vi "DC Motor Control V1.vi"() -> ()   [LabVIEW 2013, in "LabVIEW Interface for Arduino.lvlib"]
doc: "An example that reads a user selectable analog input pin on the Arduino."
uses:
  <vilib>/LabVIEW Interface for Arduino/LabVIEW Interface for Arduino.lvlib
  <vilib>/LabVIEW Interface for Arduino/Type Defs/Pin Mode.ctl
panel:
  in  "PWM1 Pin":u8
  in  "Stop":bool
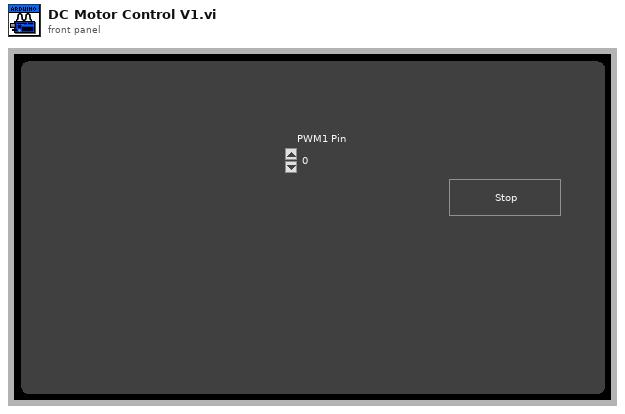
[diagram p1: front panel]
types:
  T1 = typedef "LabVIEW Interface for Arduino.lvlib/Pin Mode.ctl" = enum8{"Input", "Output"}
  T2 = typedef "LabVIEW Interface for Arduino.lvlib/Arduino Resource.ctl" = cluster{"VISA resource":refnum<visa-resource-name>, "Board Type":T3, "Connection Type":enum8{"USB / Serial"}, "Bytes Per Packet (15)":u8}
  T3 = typedef "LabVIEW Interface for Arduino.lvlib/Board Type.ctl" = enum16{"Uno", "Dimuelanove w/Atmega 328", "Mega 2560"}
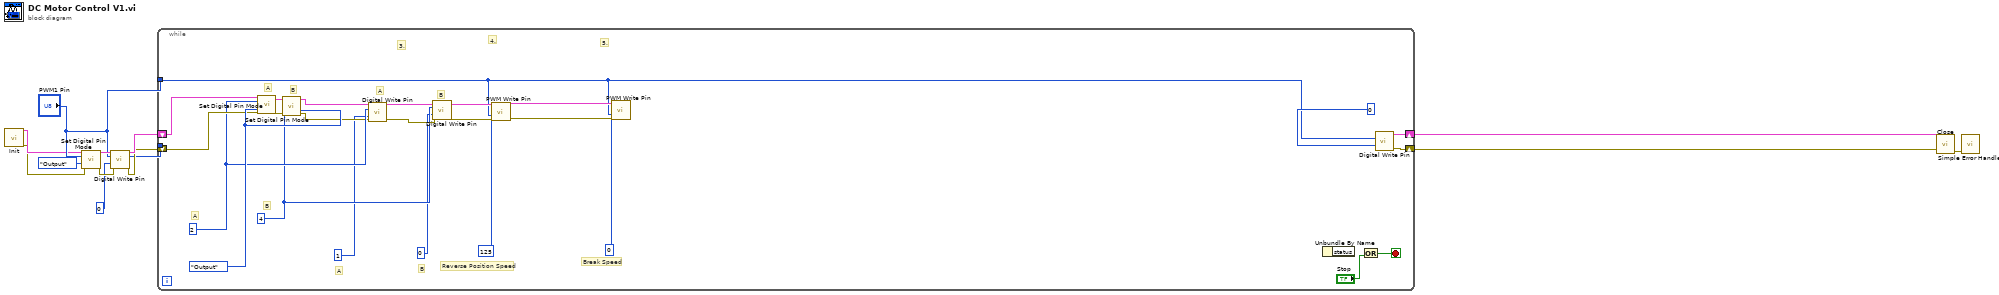
[diagram p0: block diagram]
diagram:
  n1 = call <vilib>:"Init.vi"() -> ("Arduino Resource"=w3:T2, "error out"=w2:errorcluster)  [unwired: 18 in]
  n2 = call <vilib>:"Set Digital Pin Mode.vi"("Arduino Resource"=w3, "Digital I/O Pin"="PWM1 Pin", "Pin Mode (Input)"=Pin_Mode."Output", "error in"=w2) -> ("Arduino Resource"=w9:T2, "error out"=w8:errorcluster)  [unwired: 10 in]
  n3 = call <vilib>:"Digital Write Pin.vi"("Arduino Resource"=w9, "Digital I/O Pin (0)"="PWM1 Pin", "Value (0)"=u8 0, "error in"=w8) -> ("Arduino Resource"=w6:T2, "error out"=w5:errorcluster)  [unwired: 10 in]
  n4 = while {
    shift-right: [w34] -> w11
    shift-left: w6 -> [w27]
    shift-right: [w33] -> w10
    shift-left: w5 -> [w26]
    tunnel: "PWM1 Pin" -> [_]
    tunnel: "PWM1 Pin" -> [w13]
    stop <- w37 stop-if-true
    w24 = u8 4 ("Digital I/O Pin")
    w25 = u8 2 ("Digital I/O Pin")
    w32 = Pin_Mode."Output" ("Pin Mode (Input)")
    # "Break Speed"
    # "5."
    # "4."
    # "Reverse Position Speed"
    # "3."
    # "B"
    # "A"
    # "B"
    # "A"
    # "B"
    # "A"
    # "B"
    # "A"
    n5 = call <vilib>:"Set Digital Pin Mode.vi"("Arduino Resource"=w27, "Digital I/O Pin"=w25, "Pin Mode (Input)"=w32, "error in"=w26) -> ("Arduino Resource"=w31:T2, "error out"=w30:errorcluster)  [unwired: 10 in]
    n6 = call <vilib>:"Set Digital Pin Mode.vi"("Arduino Resource"=w31, "Digital I/O Pin"=w24, "Pin Mode (Input)"=w32, "error in"=w30) -> ("Arduino Resource"=w23:T2, "error out"=w22:errorcluster)  [unwired: 10 in]
    n7 = call <vilib>:"Digital Write Pin.vi"("Arduino Resource"=w23, "Digital I/O Pin (0)"=w25, "Value (0)"=u8 1, "error in"=w22) -> ("Arduino Resource"=w29:T2, "error out"=w28:errorcluster)  [unwired: 10 in]
    n8 = call <vilib>:"Digital Write Pin.vi"("Arduino Resource"=w29, "Digital I/O Pin (0)"=w24, "Value (0)"=u8 0, "error in"=w28) -> ("Arduino Resource"=w19:T2, "error out"=w18:errorcluster)  [unwired: 10 in]
    n9 = call <vilib>:"PWM Write Pin.vi"("Arduino Resource"=w19, "Duty Cycle (0 - 255)"=u8 125, "PWM Pin (3)"=w13, "error in"=w18) -> ("Arduino Resource"=w15:T2, "error out"=w14:errorcluster)  [unwired: 10 in]
    n10 = call <vilib>:"PWM Write Pin.vi"("Arduino Resource"=w15, "Duty Cycle (0 - 255)"=u8 0, "PWM Pin (3)"=w13, "error in"=w14) -> ()  [unwired: 10 in, 2 out]
    n11 = Unbundle By Name() -> ()  [unwired: 1 in, 1 out]
    n12 = Or(y="Stop") -> (x .or. y?=w37:bool)  [unwired: 1 in]
    n13 = call <vilib>:"Digital Write Pin.vi"("Digital I/O Pin (0)"=w13, "Value (0)"=u8 0) -> ("Arduino Resource"=w34:T2, "error out"=w33:errorcluster)  [unwired: 12 in]
  }
  n14 = call <vilib>:"Close.vi"("Arduino Resource"=w11, "error in"=w10) -> ("error out"=w12:errorcluster)  [unwired: 13 in]
  n15 = call <vilib>:"Simple Error Handler.vi"("error in (no error)"=w12) -> ()  [unwired: 4 in, 5 out]
